vi "Override and Call.vi"(8 "error in (no error)":errorcluster, 11 "Override and Call Interface in":refnum<class "Override and Call Interface.lvclass">) -> (0 "error out":errorcluster, 3 "Override and Call Interface out":refnum<class "Override and Call Interface.lvclass">)   [LabVIEW 2021, in "Override and Call Interface.lvclass"]
uses:
  Override and Call Interface.lvclass
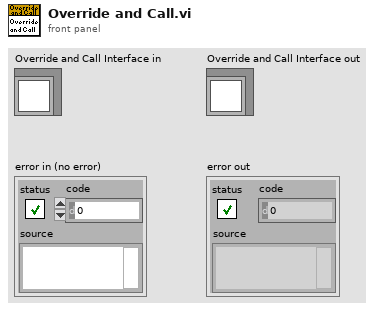
[diagram p1: front panel]
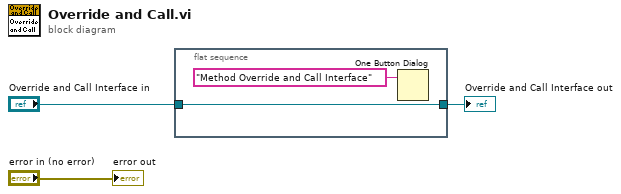
[diagram p0: block diagram]
diagram:
  n1 = flat-sequence {
    tunnel: [w4] -> w1
    tunnel: "Override and Call Interface in" -> [w4]
    frame #0 {
      n2 = One Button Dialog(message="Method Override and Call Interface") -> ()  [unwired: 1 in, 1 out]
    }
  }
  "error out" <- "error in (no error)"
  "Override and Call Interface out" <- w1
